vi "Get Ident.vi"(8 "Error In":errorcluster, 11 "reference in":refnum<class "Instrument.lvclass">) -> (0 "Error Out":errorcluster, 2 "Instr Ident":string, 3 "reference out":refnum<class "Instrument.lvclass">)   [LabVIEW 2023, in "HAL GOOP4.lvlib" / "Instrument.lvclass"]
uses:
  Instrument.lvclass
  Interfaces/IConfigure/IConfigure.lvclass
  Instrument.lvclass/Instrument.ctl
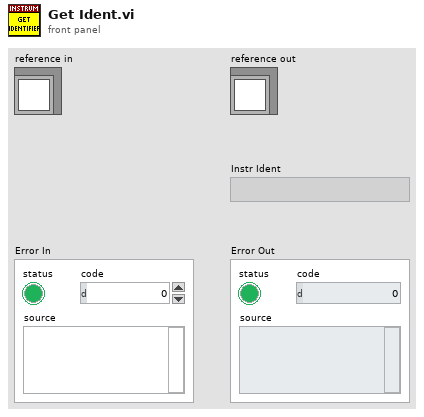
[diagram p1: front panel]
types:
  T1 = typedef "HAL GOOP4.lvlib/Instrument.lvclass/ObjectAttributes.ctl" = cluster{"IConfigure":refnum<class "IConfigure.lvclass">, "Ref Count":i16, "Start Count":i16}
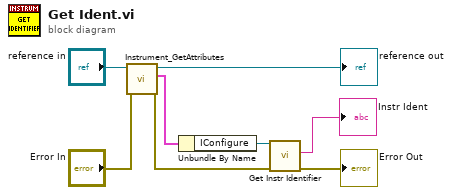
[diagram p0: block diagram]
diagram:
  n1 = call "Instrument_GetAttributes.vi"("Error In"="Error In", "reference in"="reference in") -> ("Error Out"=w7:errorcluster, "Data"=w4:T1, "reference out"=→"reference out":refnum<class "Instrument.lvclass">)  [unwired: 6 in, 1 out]
  n2 = Unbundle By Name(w4) -> ("IConfigure"=w2:refnum<class "IConfigure.lvclass">)
  n3 = call-dynamic "Get Instr Identifier.vi"("error in (no error)"=w7, "IConfigure in"=w2) -> ("error out"=→"Error Out":errorcluster, "Instr Identifier"=→"Instr Ident":string)  [unwired: 7 in, 1 out]
